vi "DetermineStartingPressureCalMultiMix.vi"(9 "Set Water Mix Pressures":dbl[](array[numeric]), 10 "New Ratio?":bool, 11 "Previous Starting Pressure":dbl[](array[numeric])) -> (2 "Starting Pressure":dbl[](array[numeric]), 3 "Which Channel To Control":enum16{"Odor Chan", "Water Chan", "Both"}(ring))   [LabVIEW 2016]
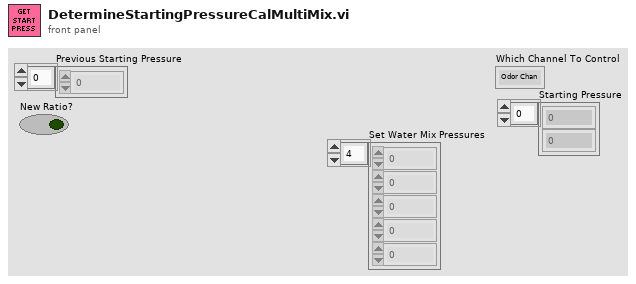
[diagram p1: front panel]
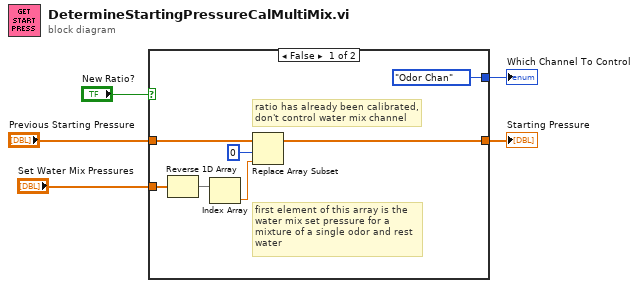
[diagram p0: block diagram]
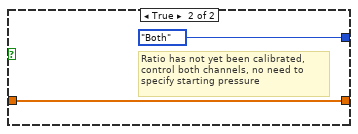
[diagram p2: hidden frame]
diagram:
  n1 = case shown="False" "New Ratio?" {
    tunnel: [enum16{"Odor Chan", "Water Chan", "Both"}."Odor Chan" ("Which Channel To Control") enum16{"Odor Chan", "Water Chan", "Both"}."Both" ("Which Channel To Control")] -> w4
    tunnel: [w9 w13] -> w2
    tunnel: "Previous Starting Pressure" -> [w11 w13]
    tunnel: "Set Water Mix Pressures" -> [w8 _]
    frame False {
      # "first element of this array is the water mix set pressure for a mixture of a single odor and rest water"
      # "ratio has already been calibrated, \ndon't control water mix channel"
      n2 = Reverse 1D Array(array=w8) -> (reversed array=w6:dbl[])
      n3 = Index Array(array=w6) -> (element=w7:dbl)  [unwired: 1 in]
      n4 = Replace Array Subset(array=w11, new element=w7, index=0) -> (w9:dbl[])
    }
    frame True {
      # "Ratio has not yet been calibrated, \ncontrol both channels, no need to specify starting pressure"
    }
  }
  "Which Channel To Control" <- w4
  "Starting Pressure" <- w2
